vi "Write I32.vi"(8 "error in (no error)":errorcluster, 9 "value":i32, 10 "Tag Name":string, 11 "Current Value Table in":refnum<class "Current Value Table.lvclass">) -> (0 "error out":errorcluster, 3 "Current Value Table out":refnum<class "Current Value Table.lvclass">)   [LabVIEW 2024, in "Current Value Table.lvlib" / "Current Value Table.lvclass"]
uses:
  Current Value Table.lvclass
  Get I32 Notifier Ref.vi
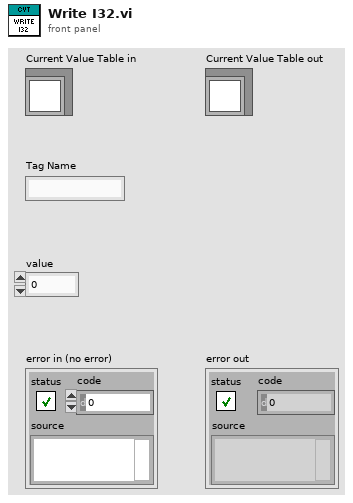
[diagram p1: front panel]
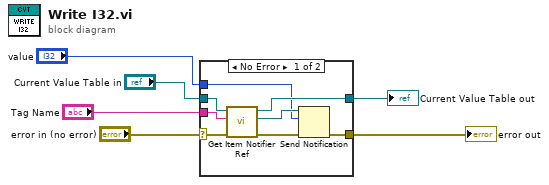
[diagram p0: block diagram]
diagram:
  n1 = case shown="No Error" "error in (no error)" {
    selector: "error in (no error)" -> [w10 w16]
    tunnel: [w14 w16] -> w5
    tunnel: [w8 w15] -> w3
    tunnel: "Current Value Table in" -> [w13 w15]
    tunnel: "Tag Name" -> [w12 _]
    tunnel: "value" -> [w7 _]
    frame No Error {
      n2 = call-poly "Get Item Notifier Ref.vi"("error in (no error)"=w10, "Tag Name"=w12, "Current Value Table in"=w13) -> ("error out"=w11:errorcluster, "notifier out"=w9:refnum<notifier>, "Current Value Table out"=w8:refnum<class "Current Value Table.lvclass">)  [unwired: 6 in]
      n3 = Send Notification(notification=w7, notifier=w9, error in (no error)=w11) -> (error out=w14:errorcluster)  [unwired: 1 out]
    }
    frame Error {
    }
  }
  "error out" <- w5
  "Current Value Table out" <- w3
